vi "Mouse Up.vi"(7 "Map Model in":refnum<class "Map Model.lvclass">, 8 "error in (no error)":errorcluster, 10 "Position":T1, 11 "Zoom In in":refnum<class "Zoom In.lvclass">) -> (0 "error out":errorcluster, 3 "Zoom In out":refnum<class "Zoom In.lvclass">, 5 "Map Model out":refnum<class "Map Model.lvclass">)   [LabVIEW 2020, in "Map Model.lvlib" / "Zoom In.lvclass"]
uses:
  Zoom In.lvclass
  E:/Project/Labview-Projects/Completed projects/Map Editor/Models/Map Model/Tools/Tool/Tool.lvclass
  <vilib>/Utility/miscctls.llb/LVPoint32TypeDef.ctl
  Map Model/Map Model.lvclass
  Tool/Tool.lvclass/Tool.ctl
  Map Model/Map Model.lvclass/Map Model.ctl
  Tool/Tool.lvclass
panel:
  # "NOTICE -- YOU MUST LEAVE THIS NOTICE IN PLACE.\n\nCopyright (c) 2017, LIANG LIU Shawn.Liu.cn@gmail.com\nAll rights reserved.\n\nRedistribution and use in source and binary forms, with or without modification, are permitted provided that the following conditions are met:\n-Redistributions of source code must retain the above copyright notice, this list of conditions and the following disclaimer.\n-Redistributions in binary form must reproduce the above copyright notice, this list of conditions and the following disclaimer in the documentation and/or other materials provided with the distribution.\n-Neither the name of the eLp nor the names of its contributors may be used to endorse or promote products derived from this software without specific prior written permission.\n\nTHIS SOFTWARE IS PROVIDED BY THE COPYRIGHT HOLDERS AND CONTRIBUTORS \"AS IS\" AND ANY EXPRESS OR IMPLIED WARRANTIES, INCLUDING, BUT NOT LIMITED TO, THE IMPLIED WARRANTIES OF MERCHANTABILITY AND FITNESS FOR A PARTICULAR PURPOSE ARE DISCLAIMED. IN NO EVENT SHALL THE COPYRIGHT HOLDER OR CONTRIBUTORS BE LIABLE FOR ANY DIRECT, INDIRECT, INCIDENTAL, SPECIAL, EXEMPLARY, OR CONSEQUENTIAL DAMAGES (INCLUDING, BUT NOT LIMITED TO, PROCUREMENT OF SUBSTITUTE GOODS OR SERVICES; LOSS OF USE, DATA, OR PROFITS; OR BUSINESS INTERRUPTION) HOWEVER CAUSED AND ON ANY THEORY OF LIABILITY, WHETHER IN CONTRACT, STRICT LIABILITY, OR TORT (INCLUDING NEGLIGENCE OR OTHERWISE) ARISING IN ANY WAY OUT OF THE USE OF THIS SOFTWARE, EVEN IF ADVISED OF THE POSSIBILITY OF SUCH DAMAGE."
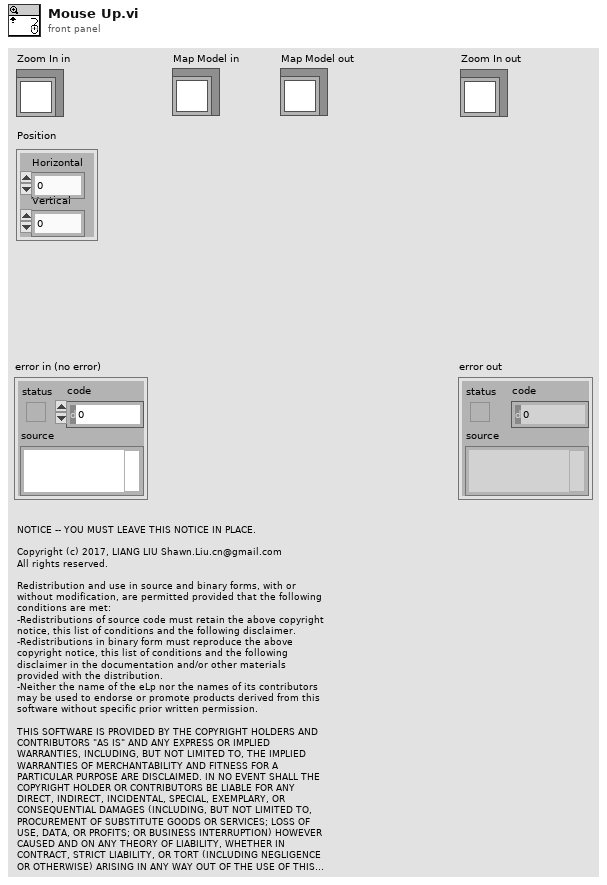
[diagram p1: front panel]
types:
  T1 = typedef "LVPoint32TypeDef.ctl" = cluster{"Horizontal":i32, "Vertical":i32}
  T2 = typedef "LVPointTypeDef.ctl" = cluster{"Horizontal":i16, "Vertical":i16}
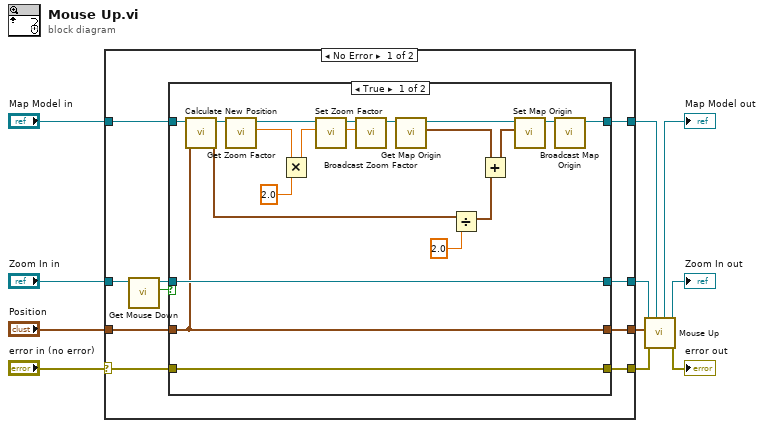
[diagram p0: block diagram]
diagram:
  n1 = case shown="No Error" "error in (no error)" {
    selector: "error in (no error)" -> [w16 w48]
    tunnel: "Zoom In in" -> [w21 w46]
    tunnel: "Map Model in" -> [w20 w47]
    tunnel: [w19 w46] -> w8
    tunnel: [w18 w47] -> w7
    tunnel: "Position" -> [w17 w45]
    tunnel: [w15 w45] -> w4
    tunnel: [w14 w48] -> w3
    frame No Error {
      n2 = call "Get Mouse Down.vi"("Tool in"=w21) -> ("Mouse Down"=w12:bool, "Tool out"=w13:refnum<class "Zoom In.lvclass">)  [unwired: 9 in]
      n3 = case shown="True" w12 {
        tunnel: w13 -> [w39 w44]
        tunnel: w20 -> [w30 w42]
        tunnel: [w31 w42] -> w18
        tunnel: [w39 w44] -> w19
        tunnel: w17 -> [w25 w41]
        tunnel: [w25 w41] -> w15
        tunnel: w16 -> [w40 w43]
        tunnel: [w40 w43] -> w14
        frame True {
          n4 = call "Calculate New Position.vi"("Position in"=w25, "Map Model in"=w30) -> ("Position out"=w24:T1, "Map Model out"=w26:refnum<class "Map Model.lvclass">)  [unwired: 8 in]
          n5 = call "Get Zoom Factor.vi"("Map Model in"=w26) -> ("Zoom Factor"=w37:dbl, "Map Model out"=w33:refnum<class "Map Model.lvclass">)  [unwired: 9 in]
          n6 = Multiply(x=w37, y=2.0 ("x")) -> (x*y=w35:dbl)
          n7 = call "Set Zoom Factor.vi"("Zoom Factor"=w35, "Map Model in"=w33) -> ("Map Model out"=w34:refnum<class "Map Model.lvclass">)  [unwired: 9 in]
          n8 = call "Broadcast Zoom Factor.vi"("Zoom Factor"=w35, "Map Model in"=w34) -> ("Map Model out"=w32:refnum<class "Map Model.lvclass">)  [unwired: 8 in, 1 out]
          n9 = call "Get Map Origin.vi"("Map Model in"=w32) -> ("Map Origin"=w23:T2, "Map Model out"=w29:refnum<class "Map Model.lvclass">)  [unwired: 9 in]
          n10 = Divide(x=w24, y=sgl 2.0 ("Zoom Factor")) -> (x/y=w28:cluster{"Horizontal":sgl, "Vertical":sgl})
          n11 = Add(x=w23, y=w28) -> (x+y=w22:cluster{"Horizontal":sgl, "Vertical":sgl})
          n12 = call "Set Map Origin.vi"("Map Origin"=w22, "Map Model in"=w29) -> ("Map Model out"=w36:refnum<class "Map Model.lvclass">)  [unwired: 9 in]
          n13 = call "Broadcast Map Origin.vi"("Map Model in"=w36) -> ("Map Model out"=w31:refnum<class "Map Model.lvclass">)  [unwired: 9 in, 1 out]
        }
        frame False {
        }
      }
    }
    frame Error {
    }
  }
  n14 = call-parent "Mouse Up.vi"("Map Model in"=w7, "error in (no error)"=w3, "Position"=w4, "Tool in"=w8) -> ("error out"=→"error out":errorcluster, "Tool out"=→"Zoom In out":refnum<class "Zoom In.lvclass">, "Map Model out"=→"Map Model out":refnum<class "Map Model.lvclass">)  [unwired: 5 in]
